vi "TDPRobotCode.vi"(0 "Sensor 1 Mode":dbl, 1 "Sensor 1 Value":dbl, 2 "Sensor 2 Mode":dbl, 3 "Sensor 2 Value":dbl) -> (15 "Motor 1 Value":dbl, 16 "Motor On Duration":dbl, 18 "Motor 2 Value":dbl)   [LabVIEW 2016]
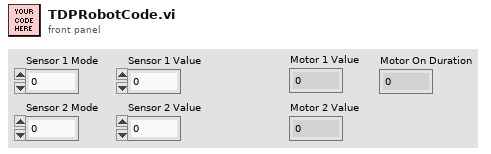
[diagram p1: front panel]
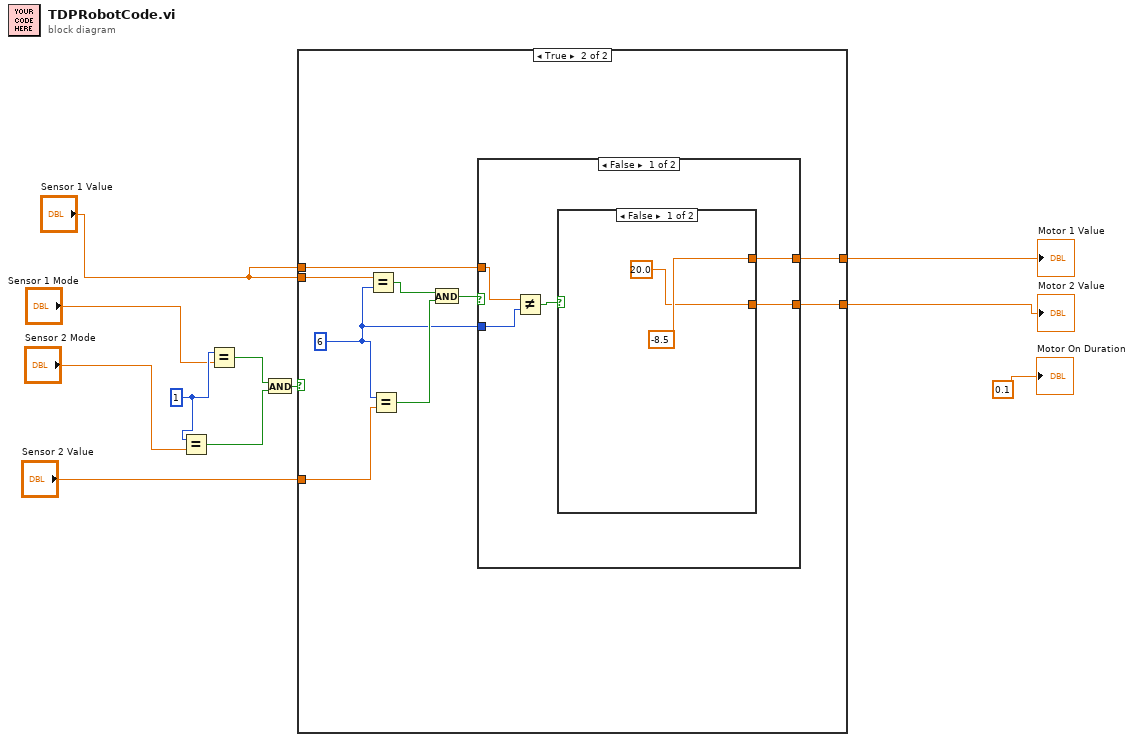
[diagram p0: block diagram]
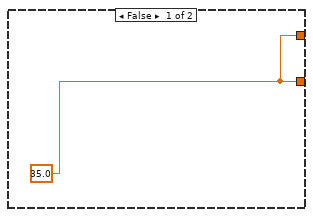
[diagram p2: hidden frame]
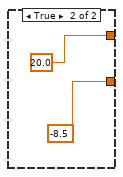
[diagram p3: hidden frame]
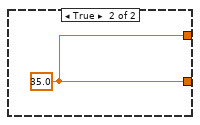
[diagram p4: hidden frame]
diagram:
  w6 = 1
  n1 = Equal?(x=w6, y="Sensor 2 Mode") -> (x = y?=w8:bool)
  n2 = Equal?(x=w6, y="Sensor 1 Mode") -> (x = y?=w9:bool)
  n3 = And(x=w9, y=w8) -> (x .and. y?=w10:bool)
  n4 = case shown="True" w10 {
    tunnel: "Sensor 1 Value" -> [_ w21]
    tunnel: "Sensor 2 Value" -> [_ w20]
    tunnel: [w12 w16] -> w3
    tunnel: [w12 w15] -> w2
    tunnel: "Sensor 1 Value" -> [_ w14]
    frame False {
      w12 = 35.0
    }
    frame True {
      w13 = 6
      n5 = Equal?(x=w21, y=w13) -> (x = y?=w19:bool)
      n6 = Equal?(x=w13, y=w20) -> (x = y?=w18:bool)
      n7 = And(x=w19, y=w18) -> (x .and. y?=w17:bool)
      n8 = case shown="False" w17 {
        tunnel: [w23 w31] -> w16
        tunnel: [w22 w31] -> w15
        tunnel: w14 -> [w25 _]
        tunnel: w13 -> [w24 _]
        frame False {
          n9 = Not Equal?(x=w25, y=w24) -> (x != y?=w26:bool)
          n10 = case shown="False" w26 {
            tunnel: [-8.5 20.0] -> w23
            tunnel: [20.0 -8.5] -> w22
            frame False {
            }
            frame True {
            }
          }
        }
        frame True {
          w31 = 35.0
        }
      }
    }
  }
  "Motor 1 Value" <- w3
  "Motor 2 Value" <- w2
  "Motor On Duration" <- 0.1
